vi "set_trajectory.vi"(8 "error in (no error)":errorcluster, 10 "trajectory":refnum<class "GenericTrajectory.lvclass">, 11 "GenericScanHead.lvclass in":refnum<class "GenericScanHead.lvclass">) -> (0 "error out":errorcluster, 3 "GenericScanHead.lvclass out":refnum<class "GenericScanHead.lvclass">)   [LabVIEW 2010, in "GenericScanHead.lvclass"]
uses:
  GenericScanHead.lvclass
  Trajectory/GenericTrajectory/GenericTrajectory/GenericTrajectory.lvclass
  GenericScanHead.lvclass/GenericScanHead.ctl
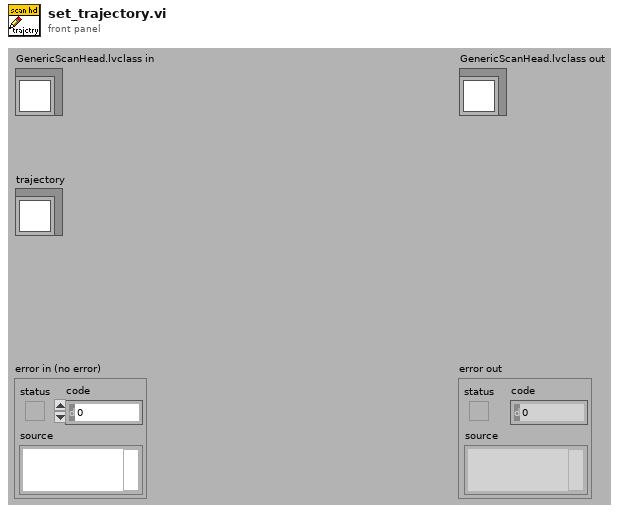
[diagram p1: front panel]
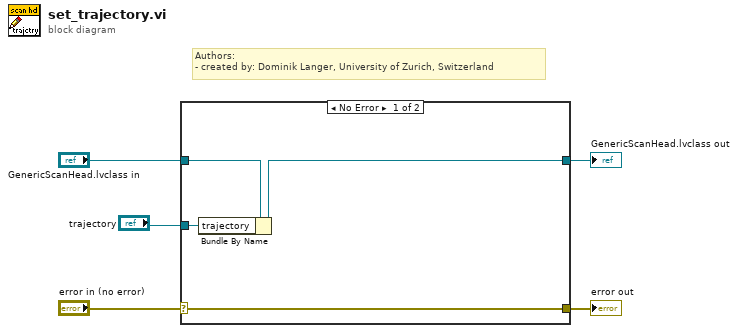
[diagram p0: block diagram]
diagram:
  # "Authors: \n- created by: Dominik Langer, University of Zurich, Switzerland"
  n1 = case shown="No Error" "error in (no error)" {
    selector: "error in (no error)" -> [w9 w10]
    tunnel: [w9 w10] -> w4
    tunnel: [w7 w11] -> w2
    tunnel: "GenericScanHead.lvclass in" -> [w8 w11]
    tunnel: "trajectory" -> [w6 _]
    frame No Error {
      n2 = Bundle By Name(cluster=w8, "trajectory"=w6) -> (w7:refnum<class "GenericScanHead.lvclass">)
    }
    frame Error {
    }
  }
  "error out" <- w4
  "GenericScanHead.lvclass out" <- w2
